vi "例5_总线操作.vi"() -> ()   [LabVIEW 2012]
panel:
  in  "使能关":bool
  out "轴状态机":string
  out "轴控制字":string
  out "轴状态字":string
  out "轴错误码":string
  out "轴类型":string
  out "轴子地址ID":string
  in  "使能开":bool
  out "轴地址ID":string
  in  "轴号：":u16
  in  "值 16#":string
  in  "长度":u16
  in  "主索引 16#":u16 format="%x"
  in  "子索引 16#":u16 format="%x"
  in  "从站ID":u16
  in  "写入参数":bool
  in  "读取参数":bool
  out "轴数":u32
  out "从站总数":u16
  out "本地输出IO数":u16
  out "本地输入IO数":u16
  out "模块输入IO数":u16
  out "模块输出IO数":u16
  out "模块DA数":u16
  out "模块AD数":u16
  in  "硬复位":bool
  in  "软复位":bool
  out "复位提示":string
  out "总线状态":string
  out "当前速度":dbl
  in  "退出":bool
  in  "卡号":u16
  # "轴信息"
  # "对象字典操作"
  # "总线状态及复位操作"
  # "从站信息"
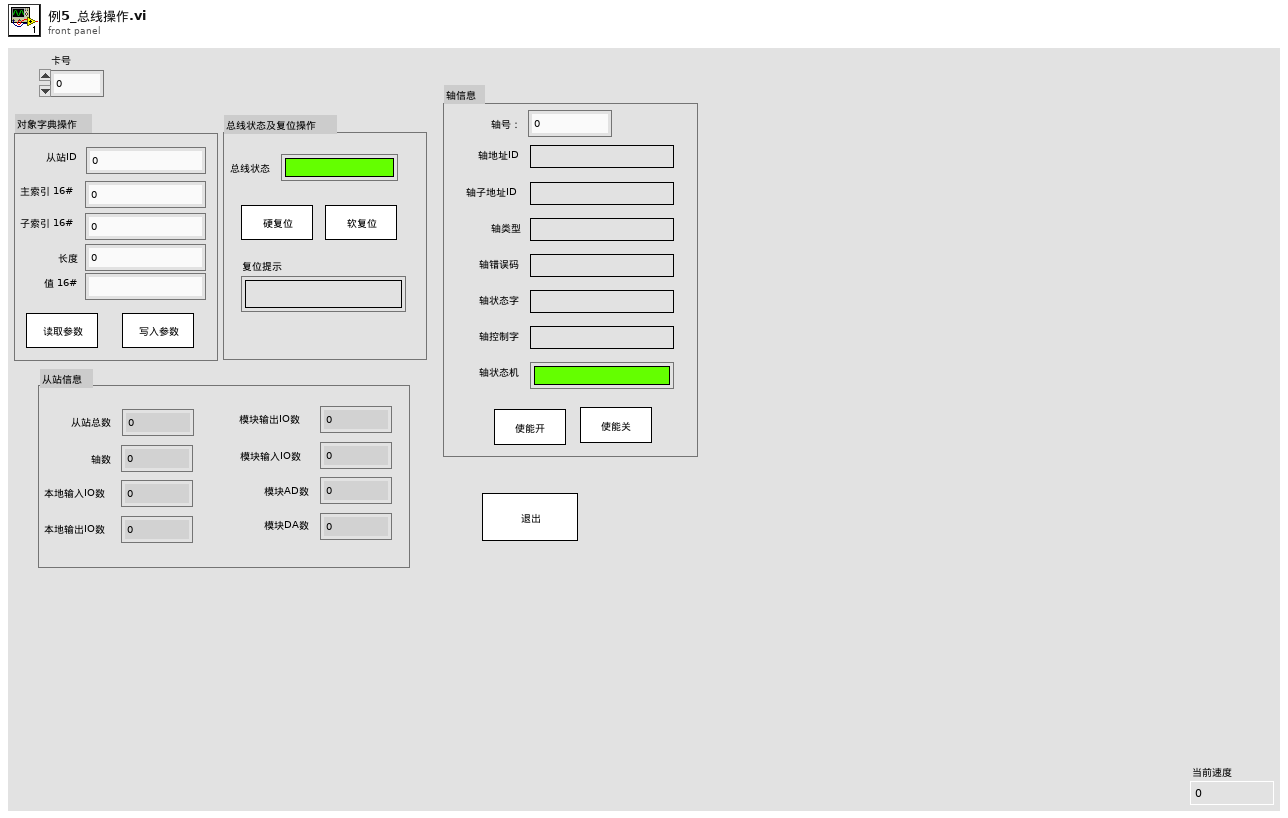
[diagram p1: front panel]
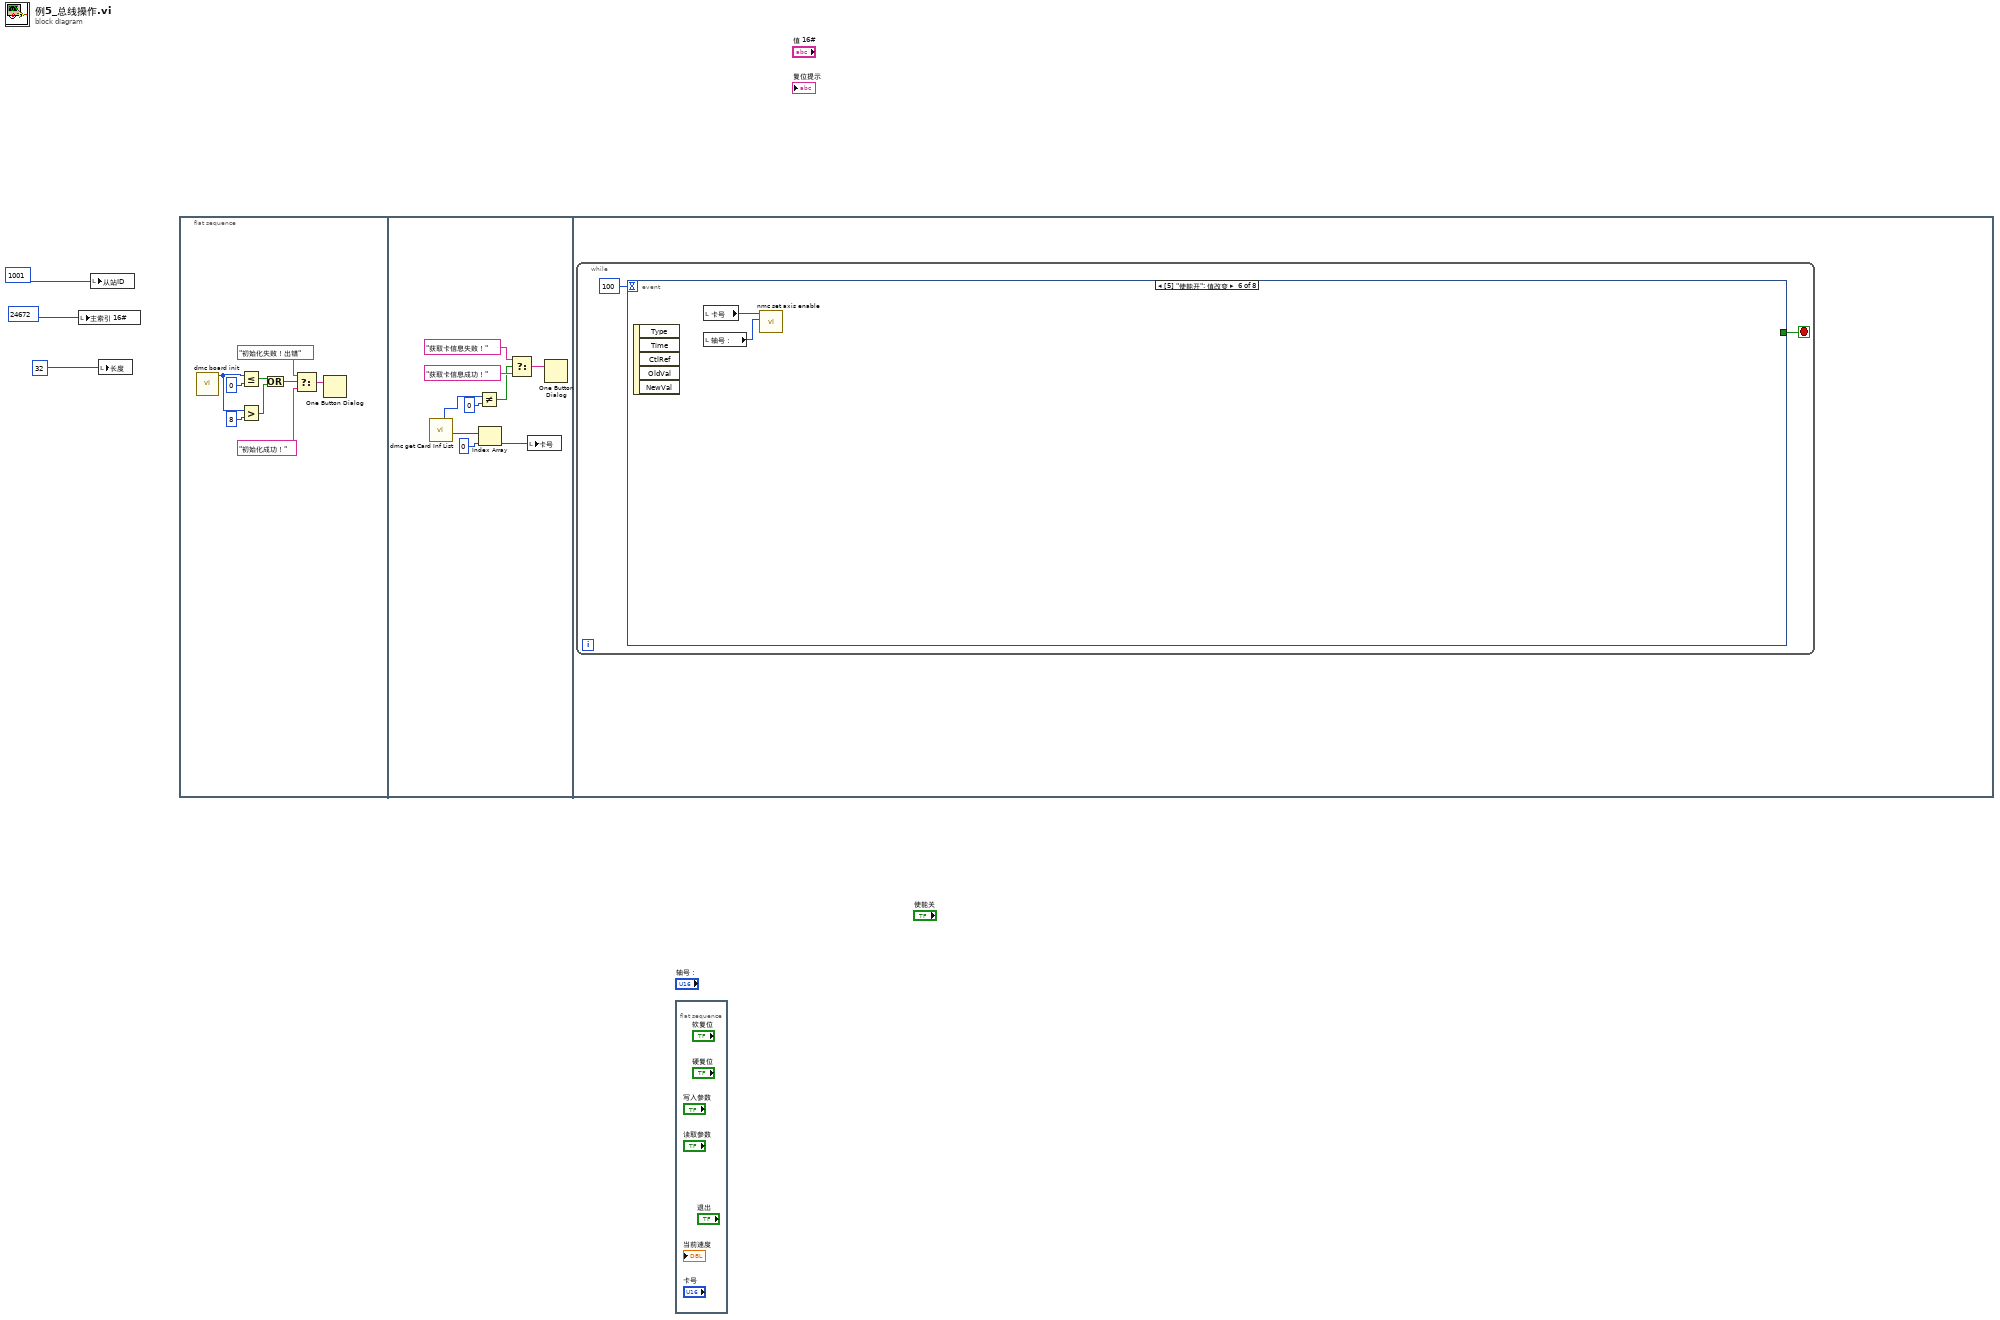
[diagram p0: block diagram]
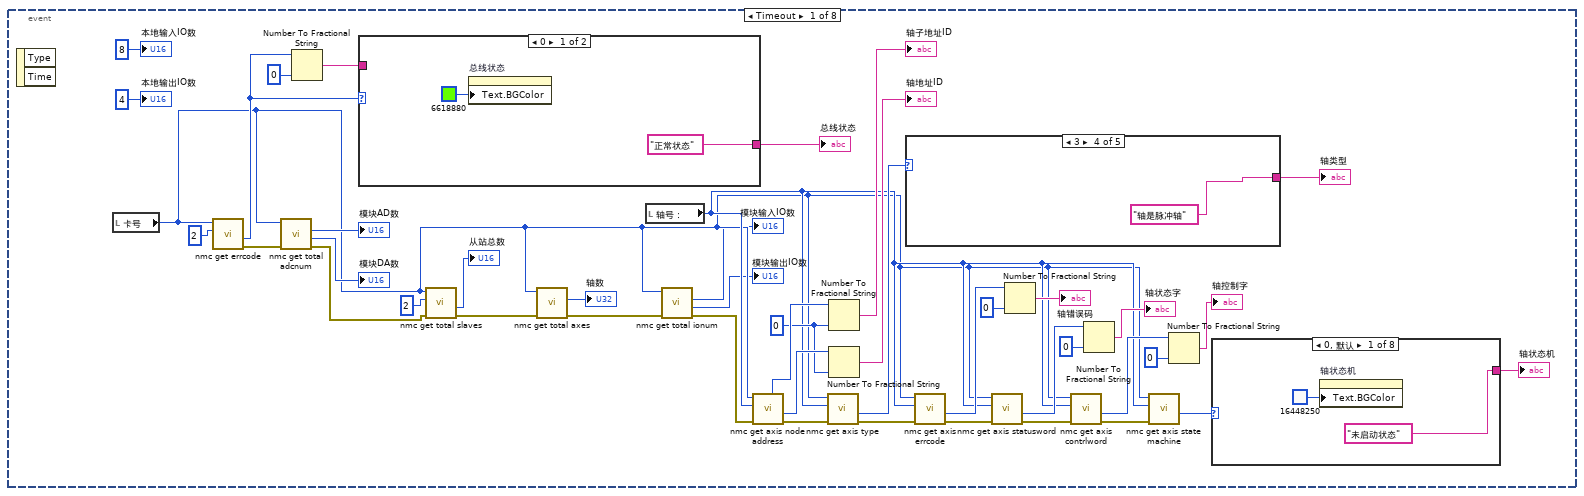
[diagram p2: hidden frame]
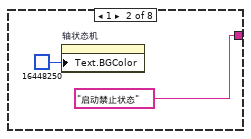
[diagram p3: hidden frame]
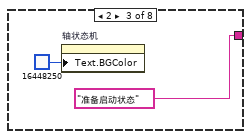
[diagram p4: hidden frame]
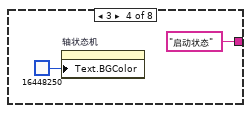
[diagram p5: hidden frame]
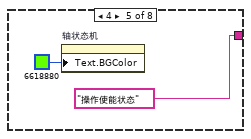
[diagram p6: hidden frame]
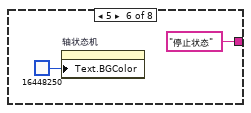
[diagram p7: hidden frame]
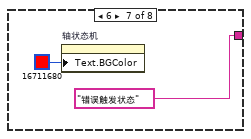
[diagram p8: hidden frame]
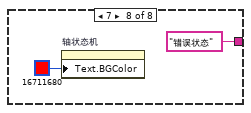
[diagram p9: hidden frame]
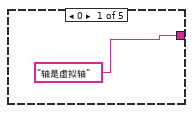
[diagram p10: hidden frame]
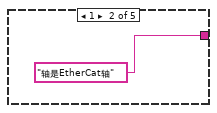
[diagram p11: hidden frame]
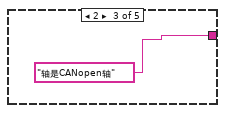
[diagram p12: hidden frame]
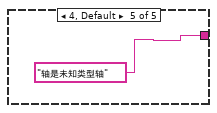
[diagram p13: hidden frame]
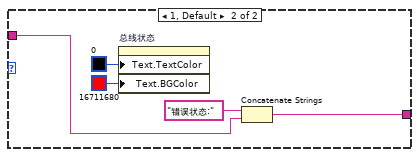
[diagram p14: hidden frame]
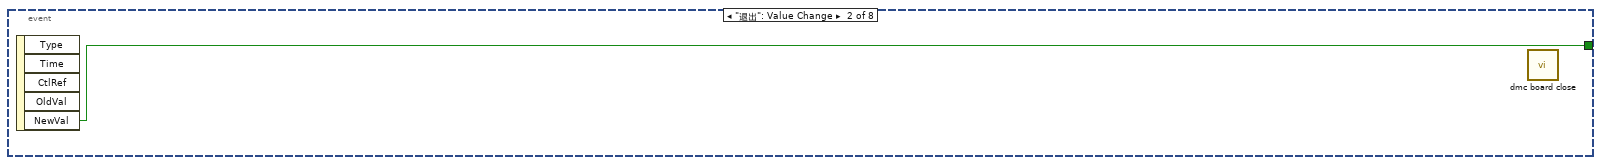
[diagram p15: hidden frame]
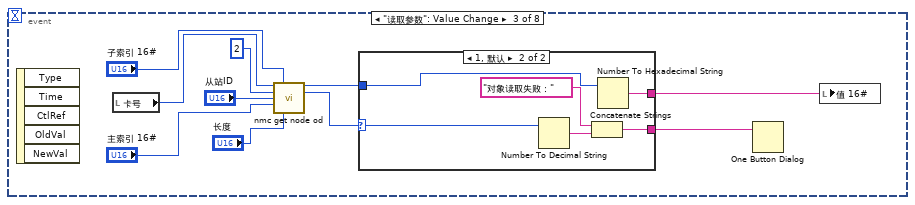
[diagram p16: hidden frame]
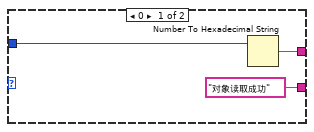
[diagram p17: hidden frame]
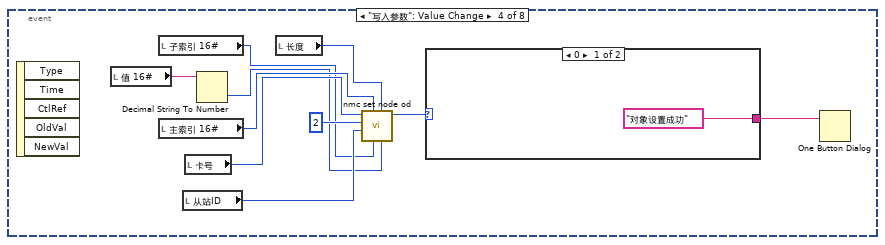
[diagram p18: hidden frame]
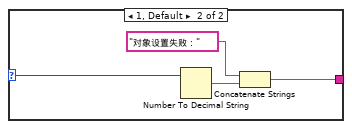
[diagram p19: hidden frame]
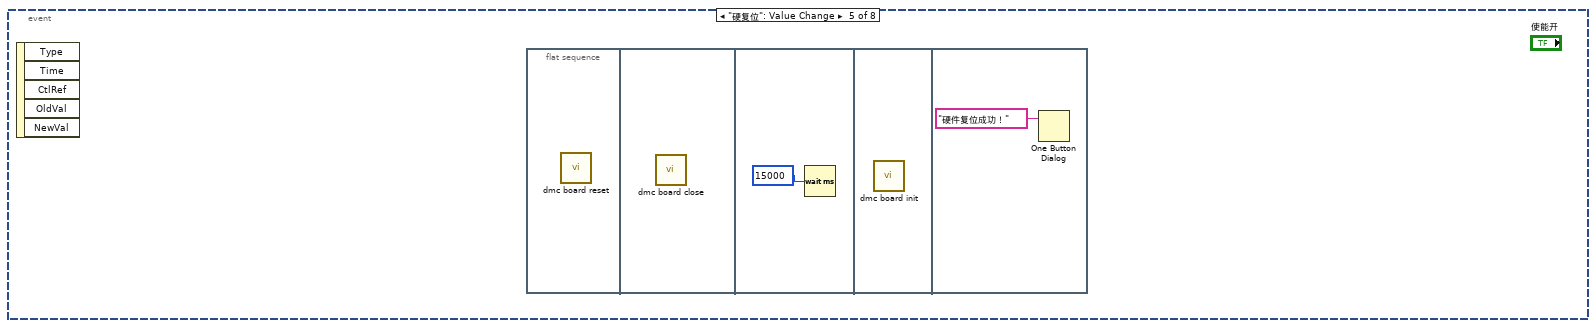
[diagram p20: hidden frame]
diagram:
  n1 = local write "主索引 16#"(24672) -> ()
  n2 = local write "从站ID"(1001) -> ()
  n3 = local write "长度"(32) -> ()
  n4 = flat-sequence {
    frame #0 {
      n5 = call "dmc board init.vi"() -> ("function return"=w5:i16)  [unwired: 10 in, 1 out]
      n6 = Less Or Equal?(x=w5, y=0) -> (x <= y?=w8:bool)
      n7 = Greater?(x=w5, y=8) -> (0:w7:bool)
      n8 = Or(x=w8, y=w7) -> (x .or. y?=w9:bool)
      n9 = Select(t="初始化失败！出错", s=w9, f="初始化成功！") -> (s? t:f=w11:string)
      n10 = One Button Dialog(message=w11) -> ()  [unwired: 1 in, 1 out]
    }
    frame #1 {
      n11 = call "dmc get Card Inf List.vi"() -> ("CardIdList out"=w15:u16[], "function return"=w16:i16)  [unwired: 7 in, 3 out]
      n12 = Not Equal?(x=w16, y=0) -> (x != y?=w18:bool)
      n13 = Index Array(array=w15, index=0) -> (element=w13:u16)
      n14 = Select(t="获取卡信息失败！", s=w18, f="获取卡信息成功！") -> (s? t:f=w21:string)
      n15 = local write "卡号"(w13) -> ()
      n16 = One Button Dialog(message=w21) -> ()  [unwired: 1 in, 1 out]
    }
    frame #2 {
      n17 = while {
        stop <- w23 stop-if-true
        n18 = event shown="[5] \"使能开\": 值改变" {
          selector: _ -> [_ _ _ _ _ _ _ _]
          dyn-events: _ -> [_ _ _ _ _ _ _ _]
          timeout: 100 -> [_ _ _ _ _ _ _ _]
          tunnel: [_ w96 _ _ _ _ _ _] -> w23
          event Timeout {
            w58 = i16 0 ("精度(6)")
            n19 = event-data() -> ()  [unwired: 1 in, 2 out]
            n20 = local read "卡号"() -> (w29:u16)
            n21 = call "nmc get errcode.vi"("channel"=u16 2, "CardNo"=w29) -> ("error out"=w34:errorcluster, "Errcode out"=w64:u16)  [unwired: 7 in, 1 out]
            n22 = call "nmc get total adcnum.vi"("error in (no error)"=w34, "CardNo"=w29) -> ("error out"=w33:errorcluster, "TotalOut out"=→"模块DA数":u16, "TotalIn out"=→"模块AD数":u16)  [unwired: 6 in, 1 out]
            n23 = Number To Fractional String(number=w64, precision (6)=i16 0 ("精度(6)")) -> (F-format string=w63:string)  [unwired: 2 in]
            n24 = case shown="0" w64 {
              tunnel: ["正常状态" ("轴状态机") w93] -> w67
              tunnel: w63 -> [_ w94]
              frame 0 {
                n25 = property on="总线状态" class="Str"("Text.BGColor"=u32 6618880) -> ()  [unwired: 2 in, 2 out]
              }
              frame 1, Default {
                n26 = property on="总线状态" class="Str"("Text.TextColor"=u32 0, "Text.BGColor"=u32 16711680) -> ()  [unwired: 2 in, 2 out]
                n27 = Concatenate Strings("错误状态:" ("轴状态机"), w94) -> (w93:string)
              }
            }
            "总线状态" <- w67
            n28 = call "nmc get total slaves.vi"("error in (no error)"=w33, "PortNum"=u16 2, "CardNo"=w29) -> ("error out"=w32:errorcluster, "TotalSlaves out"=→"从站总数":u16)  [unwired: 6 in, 1 out]
            n29 = call "nmc get total axes.vi"("error in (no error)"=w32, "CardNo"=w29) -> ("error out"=w30:errorcluster, "TotalAxis out"=→"轴数":u32)  [unwired: 7 in, 1 out]
            n30 = local read "轴号："() -> (w39:u16)
            n31 = call "nmc get total ionum.vi"("error in (no error)"=w30, "CardNo"=w29) -> ("error out"=w24:errorcluster, "TotalOut out"=→"模块输出IO数":u16, "TotalIn out"=→"模块输入IO数":u16)  [unwired: 6 in, 1 out]
            n32 = call "nmc get axis node address.vi"("error in (no error)"=w24, "axis"=w39, "CardNo"=w29) -> ("error out"=w53:errorcluster, "SlaveAddr out"=w59:u16, "Sub_SlaveAddr out"=w60:u16)  [unwired: 5 in, 1 out]
            n33 = call "nmc get axis type.vi"("error in (no error)"=w53, "axis"=w39, "CardNo"=w29) -> ("error out"=w52:errorcluster, "Axis_Type out"=w55:u16)  [unwired: 6 in, 1 out]
            n34 = Number To Fractional String(number=w60, precision (6)=w58) -> (F-format string=→"轴子地址ID":string)  [unwired: 2 in]
            n35 = Number To Fractional String(number=w59, precision (6)=w58) -> (F-format string=→"轴地址ID":string)  [unwired: 2 in]
            n36 = case shown="3" w55 {
              tunnel: ["轴是虚拟轴" ("F-格式字符串") "轴是EtherCat轴" ("F-格式字符串") "轴是CANopen轴" ("F-格式字符串") "轴是脉冲轴" ("F-格式字符串") "轴是未知类型轴" ("F-格式字符串")] -> w54
              frame 0 {
              }
              frame 1 {
              }
              frame 2 {
              }
              frame 3 {
              }
              frame 4, Default {
              }
            }
            "轴类型" <- w54
            n37 = call "nmc get axis errcode.vi"("error in (no error)"=w52, "axis"=w39, "CardNo"=w29) -> ("error out"=w48:errorcluster, "Errcode out"=w51:u16)  [unwired: 6 in, 1 out]
            n38 = call "nmc get axis statusword.vi"("error in (no error)"=w48, "axis"=w39, "CardNo"=w29) -> ("error out"=w41:errorcluster, "statusword out"=w46:i32)  [unwired: 6 in, 1 out]
            n39 = Number To Fractional String(number=w51, precision (6)=i16 0 ("精度(6)")) -> (F-format string=→"轴错误码":string)  [unwired: 2 in]
            n40 = call "nmc get axis contrlword.vi"("error in (no error)"=w41, "Axis"=w39, "CardNo"=w29) -> ("error out"=w40:errorcluster, "Contrlword out"=w43:i32)  [unwired: 6 in, 1 out]
            n41 = Number To Fractional String(number=w46, precision (6)=i16 0 ("精度(6)")) -> (F-format string=→"轴状态字":string)  [unwired: 2 in]
            n42 = call "nmc get axis state machine.vi"("error in (no error)"=w40, "axis"=w39, "CardNo"=w29) -> ("Axis_StateMachine out"=w38:u16)  [unwired: 6 in, 2 out]
            n43 = Number To Fractional String(number=w43, precision (6)=i16 0 ("精度(6)")) -> (F-format string=→"轴控制字":string)  [unwired: 2 in]
            n44 = case shown="0, 默认" w38 {
              tunnel: ["未启动状态" ("轴状态机") "启动禁止状态" ("轴状态机") "准备启动状态" ("轴状态机") "启动状态" ("轴状态机") "操作使能状态" ("轴状态机") "停止状态" ("轴状态机") "错误触发状态" ("轴状态机") "错误状态" ("轴状态机")] -> w37
              frame 0, Default {
                n45 = property on="轴状态机" class="Str"("Text.BGColor"=u32 16448250) -> ()  [unwired: 2 in, 2 out]
              }
              frame 1 {
                n46 = property on="轴状态机" class="Str"("Text.BGColor"=u32 16448250) -> ()  [unwired: 2 in, 2 out]
              }
              frame 2 {
                n47 = property on="轴状态机" class="Str"("Text.BGColor"=u32 16448250) -> ()  [unwired: 2 in, 2 out]
              }
              frame 3 {
                n48 = property on="轴状态机" class="Str"("Text.BGColor"=u32 16448250) -> ()  [unwired: 2 in, 2 out]
              }
              frame 4 {
                n49 = property on="轴状态机" class="Str"("Text.BGColor"=u32 6618880) -> ()  [unwired: 2 in, 2 out]
              }
              frame 5 {
                n50 = property on="轴状态机" class="Str"("Text.BGColor"=u32 16448250) -> ()  [unwired: 2 in, 2 out]
              }
              frame 6 {
                n51 = property on="轴状态机" class="Str"("Text.BGColor"=u32 16711680) -> ()  [unwired: 2 in, 2 out]
              }
              frame 7 {
                n52 = property on="轴状态机" class="Str"("Text.BGColor"=u32 16711680) -> ()  [unwired: 2 in, 2 out]
              }
            }
            "轴状态机" <- w37
            "本地输入IO数" <- u16 8 ("本地输入IO数")
            "本地输出IO数" <- u16 4 ("本地输出IO数")
          }
          event "退出": Value Change {
            n53 = event-data() -> ("NewVal"=w96:bool)  [unwired: 1 in, 4 out]
            n54 = call "dmc board close.vi"() -> ()  [unwired: 10 in, 2 out]
          }
          event "读取参数": Value Change {
            n55 = event-data() -> ()  [unwired: 1 in, 5 out]
            n56 = local read "卡号"() -> (w106:u16)
            n57 = call "nmc get node od.vi"("CardNo"=w106, "SubIndex"="子索引 16#", "PortNum"=u16 2, "NodeNum"="从站ID", "Index"="主索引 16#", "ValLength"="长度") -> ("Value out"=w98:i32, "function return"=w99:i16)  [unwired: 7 in, 1 out]
            n58 = case shown="1, 默认" w99 {
              selector: w99 -> [_ w113]
              tunnel: ["对象读取成功" ("消息") w114] -> w100
              tunnel: w98 -> [w108 w110]
              tunnel: [w107 w111] -> w97
              frame 0 {
                n59 = Number To Hexadecimal String(2:w108) -> (0:w107:string)  [unwired: 1 in]
              }
              frame 1, Default {
                n60 = Number To Decimal String(number=w113) -> (decimal integer string=w112:string)  [unwired: 1 in]
                n61 = Concatenate Strings("对象读取失败：" ("消息"), w112) -> (w114:string)
                n62 = Number To Hexadecimal String(2:w110) -> (0:w111:string)  [unwired: 1 in]
              }
            }
            n63 = One Button Dialog(message=w100) -> ()  [unwired: 1 in, 1 out]
            n64 = local write "值 16#"(w97) -> ()
          }
          event "写入参数": Value Change {
            n65 = event-data() -> ()  [unwired: 1 in, 5 out]
            n66 = local read "值 16#"() -> (w119:string)
            n67 = local read "子索引 16#"() -> (w121:u16)
            n68 = local read "主索引 16#"() -> (w122:u16)
            n69 = local read "从站ID"() -> (w123:u16)
            n70 = local read "卡号"() -> (w125:u16)
            n71 = Decimal String To Number(string=w119) -> (number=w118:i32)  [unwired: 2 in, 1 out]
            n72 = local read "长度"() -> (w120:u16)
            n73 = call "nmc set node od.vi"("Value"=w118, "ValLength"=w120, "SubIndex"=w121, "Index"=w122, "NodeNum"=w123, "PortNum"=u16 2, "CardNo"=w125) -> ("function return"=w116:i16)  [unwired: 3 in, 1 out]
            n74 = case shown="0" w116 {
              selector: w116 -> [_ w128]
              tunnel: ["对象设置成功" ("消息") w129] -> w117
              frame 0 {
              }
              frame 1, Default {
                n75 = Number To Decimal String(number=w128) -> (decimal integer string=w127:string)  [unwired: 1 in]
                n76 = Concatenate Strings("对象设置失败：" ("消息"), w127) -> (w129:string)
              }
            }
            n77 = One Button Dialog(message=w117) -> ()  [unwired: 1 in, 1 out]
          }
          event "硬复位": Value Change {
            n78 = event-data() -> ()  [unwired: 1 in, 5 out]
            n79 = flat-sequence {
              frame #0 {
                n80 = call "dmc board reset.vi"() -> ()  [unwired: 10 in, 2 out]
              }
              frame #1 {
                n81 = call "dmc board close.vi"() -> ()  [unwired: 10 in, 2 out]
              }
              frame #2 {
                n82 = Wait (ms)(milliseconds to wait=15000) -> ()  [unwired: 1 out]
              }
              frame #3 {
                n83 = call "dmc board init.vi"() -> ()  [unwired: 10 in, 2 out]
              }
              frame #4 {
                n84 = One Button Dialog(message="硬件复位成功！") -> ()  [unwired: 1 in, 1 out]
              }
            }
          }
          event "使能开": Value Change {
            n85 = event-data() -> ()  [unwired: 1 in, 5 out]
            n86 = local read "卡号"() -> (w134:u16)
            n87 = local read "轴号："() -> (w133:u16)
            n88 = call "nmc set axis enable.vi"("axis"=w133, "CardNo"=w134) -> ()  [unwired: 8 in, 2 out]
          }
          event "使能关": Value Change {
            n89 = event-data() -> ()  [unwired: 1 in, 5 out]
            n90 = local read "轴号："() -> (w135:u16)
            n91 = local read "卡号"() -> (w136:u16)
            n92 = call "nmc set axis disable.vi"("axis"=w135, "CardNo"=w136) -> ()  [unwired: 8 in, 2 out]
          }
          event "软复位": Value Change {
            n93 = event-data() -> ()  [unwired: 1 in, 5 out]
            n94 = flat-sequence {
              frame #0 {
                n95 = local read "卡号"() -> (w137:u16)
                n96 = call "dmc soft reset.vi"("CardNo"=w137) -> ()  [unwired: 9 in, 2 out]
              }
              frame #1 {
                n97 = call "dmc board close.vi"() -> ()  [unwired: 10 in, 2 out]
              }
              frame #2 {
                n98 = Wait (ms)(milliseconds to wait=15000) -> ()  [unwired: 1 out]
              }
              frame #3 {
                n99 = call "dmc board init.vi"() -> ()  [unwired: 10 in, 2 out]
              }
              frame #4 {
                n100 = One Button Dialog(message="软件复位成功！") -> ()  [unwired: 1 in, 1 out]
              }
            }
          }
        }
      }
    }
  }
  n101 = flat-sequence {
    frame #0 {
    }
  }
